vi "segment function.vi"(4 "y2":dbl, 5 "y1":dbl, 6 "x2":dbl, 7 "x1":dbl, 11 "x":dbl) -> (3 "y":dbl)   [LabVIEW 2023]
panel:
  # "0<=x<=1, same for x1, x2"
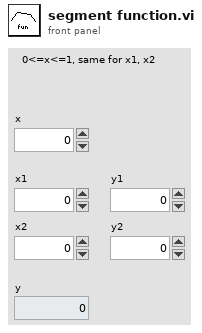
[diagram p1: front panel]
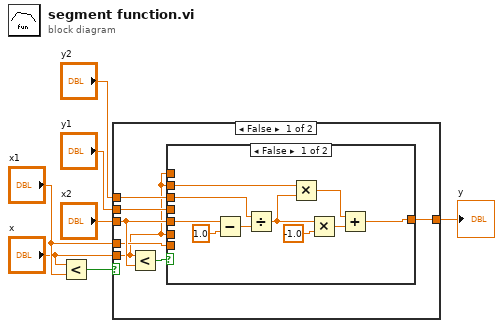
[diagram p0: block diagram]
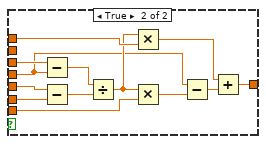
[diagram p2: hidden frame]
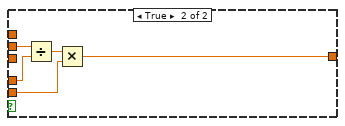
[diagram p3: hidden frame]
diagram:
  n1 = Less?(x="x", y="x1") -> (x < y?=w7:bool)
  n2 = case shown="False" w7 {
    tunnel: "x1" -> [w10 w42]
    tunnel: "y1" -> [w12 w41]
    tunnel: "x" -> [w8 w39]
    tunnel: [w9 w38] -> w3
    tunnel: "x2" -> [w11 _]
    tunnel: "y2" -> [w13 _]
    frame False {
      n3 = Less?(x=w8, y=w11) -> (x < y?=w14:bool)
      n4 = case shown="False" w14 {
        tunnel: w13 -> [w20 w37]
        tunnel: w12 -> [_ w28]
        tunnel: w11 -> [w23 w35]
        tunnel: w8 -> [_ w34]
        tunnel: w8 -> [_ w32]
        tunnel: w10 -> [_ w29]
        tunnel: [w15 w25] -> w9
        tunnel: w8 -> [w24 _]
        frame False {
          n5 = Subtract(x=w23, y=1.0) -> (x-y=w21:dbl)
          n6 = Divide(x=w20, y=w21) -> (x/y=w18:dbl)
          n7 = Multiply(x=w24, y=w18) -> (x*y=w19:dbl)
          n8 = Multiply(x=w18, y=-1.0) -> (x*y=w16:dbl)
          n9 = Add(x=w19, y=w16) -> (x+y=w15:dbl)
        }
        frame True {
          n10 = Subtract(x=w37, y=w28) -> (x-y=w36:dbl)
          n11 = Subtract(x=w35, y=w34) -> (x-y=w33:dbl)
          n12 = Divide(x=w36, y=w33) -> (x/y=w30:dbl)
          n13 = Multiply(x=w30, y=w32) -> (x*y=w31:dbl)
          n14 = Multiply(x=w30, y=w29) -> (x*y=w27:dbl)
          n15 = Subtract(x=w28, y=w27) -> (x-y=w26:dbl)
          n16 = Add(x=w31, y=w26) -> (x+y=w25:dbl)
        }
      }
    }
    frame True {
      n17 = Divide(x=w41, y=w42) -> (x/y=w40:dbl)
      n18 = Multiply(x=w40, y=w39) -> (x*y=w38:dbl)
    }
  }
  "y" <- w3
